vi "App - analyze RUS V6.vi"() -> ()   [LabVIEW 2015] (continued)
"Magn Field(T)"=0.0}, {"temperature"=56.174, "lorentzian"={"Amplitude"=0.0, "omega(0)"=0.0, "Gamma"=0.0, "phase"=0.0, "Q"=0.0, "Norm  Ampl"=0.0, "z (inf)"=0.0+0.0i, "4corners"={"z (-pi/2)"=0.0+0.0i, "z(inf)"=0.0+0.0i, "z (pi/2)"=0.0+0.0i, "z center"=0.0+0.0i, "z(0)"=0.0+0.0i, "radius"=0.0}}, "timestamp(min)"=1312.25, "timestamp"=timestamp(3493806556 s since 1904-01-01), "Magn Field(T)"=0.0}, {"temperature"=56.114, "lorentzian"={"Amplitude"=0.0, "omega(0)"=0.0, "Gamma"=0.0, "phase"=0.0, "Q"=0.0, "Norm  Ampl"=0.0, "z (inf)"=0.0+0.0i, "4corners"={"z (-pi/2)"=0.0+0.0i, "z(inf)"=0.0+0.0i, "z (pi/2)"=0.0+0.0i, "z center"=0.0+0.0i, "z(0)"=0.0+0.0i, "radius"=0.0}}, "timestamp(min)"=1313.5666666701436, "timestamp"=timestamp(3493806635 s since 1904-01-01), "Magn Field(T)"=0.0}, {"temperature"=56.051, "lorentzian"={"Amplitude"=0.0, "omega(0)"=0.0, "Gamma"=0.0, "phase"=0.0, "Q"=0.0, "Norm  Ampl"=0.0, "z (inf)"=0.0+0.0i, "4corners"={"z (-pi/2)"=0.0+0.0i, "z(inf)"=0.0+0.0i, "z (pi/2)"=0.0+0.0i, "z center"=0.0+0.0i, "z(0)"=0.0+0.0i, "radius"=0.0}}, "timestamp(min)"=1314.8833333328366, "timestamp"=timestamp(3493806714 s since 1904-01-01), "Magn Field(T)"=0.0}, {"temperature"=55.989, "lorentzian"={"Amplitude"=0.0, "omega(0)"=0.0, "Gamma"=0.0, "phase"=0.0, "Q"=0.0, "Norm  Ampl"=0.0, "z (inf)"=0.0+0.0i, "4corners"={"z (-pi/2)"=0.0+0.0i, "z(inf)"=0.0+0.0i, "z (pi/2)"=0.0+0.0i, "z center"=0.0+0.0i, "z(0)"=0.0+0.0i, "radius"=0.0}}, "timestamp(min)"=1316.2166666686535, "timestamp"=timestamp(3493806794 s since 1904-01-01), "Magn Field(T)"=0.0}, {"temperature"=55.93, "lorentzian"={"Amplitude"=0.0, "omega(0)"=0.0, "Gamma"=0.0, "phase"=0.0, "Q"=0.0, "Norm  Ampl"=0.0, "z (inf)"=0.0+0.0i, "4corners"={"z (-pi/2)"=0.0+0.0i, "z(inf)"=0.0+0.0i, "z (pi/2)"=0.0+0.0i, "z center"=0.0+0.0i, "z(0)"=0.0+0.0i, "radius"=0.0}}, "timestamp(min)"=1317.5333333313465, "timestamp"=timestamp(3493806873 s since 1904-01-01), "Magn Field(T)"=0.0}, {"temperature"=55.865, "lorentzian"={"Amplitude"=0.0, "omega(0)"=0.0, "Gamma"=0.0, "phase"=0.0, "Q"=0.0, "Norm  Ampl"=0.0, "z (inf)"=0.0+0.0i, "4corners"={"z (-pi/2)"=0.0+0.0i, "z(inf)"=0.0+0.0i, "z (pi/2)"=0.0+0.0i, "z center"=0.0+0.0i, "z(0)"=0.0+0.0i, "radius"=0.0}}, "timestamp(min)"=1318.8500000014901, "timestamp"=timestamp(3493806952 s since 1904-01-01), "Magn Field(T)"=0.0}, {"temperature"=55.805, "lorentzian"={"Amplitude"=0.0, "omega(0)"=0.0, "Gamma"=0.0, "phase"=0.0, "Q"=0.0, "Norm  Ampl"=0.0, "z (inf)"=0.0+0.0i, "4corners"={"z (-pi/2)"=0.0+0.0i, "z(inf)"=0.0+0.0i, "z (pi/2)"=0.0+0.0i, "z center"=0.0+0.0i, "z(0)"=0.0+0.0i, "radius"=0.0}}, "timestamp(min)"=1320.183333337307, "timestamp"=timestamp(3493807032 s since 1904-01-01), "Magn Field(T)"=0.0}, {"temperature"=55.744, "lorentzian"={"Amplitude"=0.0, "omega(0)"=0.0, "Gamma"=0.0, "phase"=0.0, "Q"=0.0, "Norm  Ampl"=0.0, "z (inf)"=0.0+0.0i, "4corners"={"z (-pi/2)"=0.0+0.0i, "z(inf)"=0.0+0.0i, "z (pi/2)"=0.0+0.0i, "z center"=0.0+0.0i, "z(0)"=0.0+0.0i, "radius"=0.0}}, "timestamp(min)"=1321.5, "timestamp"=timestamp(3493807111 s since 1904-01-01), "Magn Field(T)"=0.0}, {"temperature"=55.681, "lorentzian"={"Amplitude"=0.0, "omega(0)"=0.0, "Gamma"=0.0, "phase"=0.0, "Q"=0.0, "Norm  Ampl"=0.0, "z (inf)"=0.0+0.0i, "4corners"={"z (-pi/2)"=0.0+0.0i, "z(inf)"=0.0+0.0i, "z (pi/2)"=0.0+0.0i, "z center"=0.0+0.0i, "z(0)"=0.0+0.0i, "radius"=0.0}}, "timestamp(min)"=1322.8333333358169, "timestamp"=timestamp(3493807191 s since 1904-01-01), "Magn Field(T)"=0.0}, {"temperature"=55.622, "lorentzian"={"Amplitude"=0.0, "omega(0)"=0.0, "Gamma"=0.0, "phase"=0.0, "Q"=0.0, "Norm  Ampl"=0.0, "z (inf)"=0.0+0.0i, "4corners"={"z (-pi/2)"=0.0+0.0i, "z(inf)"=0.0+0.0i, "z (pi/2)"=0.0+0.0i, "z center"=0.0+0.0i, "z(0)"=0.0+0.0i, "radius"=0.0}}, "timestamp(min)"=1324.1499999985099, "timestamp"=timestamp(3493807270 s since 1904-01-01), "Magn Field(T)"=0.0}, {"temperature"=55.56, "lorentzian"={"Amplitude"=0.0, "omega(0)"=0.0, "Gamma"=0.0, "phase"=0.0, "Q"=0.0, "Norm  Ampl"=0.0, "z (inf)"=0.0+0.0i, "4corners"={"z (-pi/2)"=0.0+0.0i, "z(inf)"=0.0+0.0i, "z (pi/2)"=0.0+0.0i, "z center"=0.0+0.0i, "z(0)"=0.0+0.0i, "radius"=0.0}}, "timestamp(min)"=1325.4666666686535, "timestamp"=timestamp(3493807349 s since 1904-01-01), "Magn Field(T)"=0.0}, {"temperature"=55.498, "lorentzian"={"Amplitude"=0.0, "omega(0)"=0.0, "Gamma"=0.0, "phase"=0.0, "Q"=0.0, "Norm  Ampl"=0.0, "z (inf)"=0.0+0.0i, "4corners"={"z (-pi/2)"=0.0+0.0i, "z(inf)"=0.0+0.0i, "z (pi/2)"=0.0+0.0i, "z center"=0.0+0.0i, "z(0)"=0.0+0.0i, "radius"=0.0}}, "timestamp(min)"=1326.8000000044703, "timestamp"=timestamp(3493807429 s since 1904-01-01), "Magn Field(T)"=0.0}, {"temperature"=55.437, "lorentzian"={"Amplitude"=0.0, "omega(0)"=0.0, "Gamma"=0.0, "phase"=0.0, "Q"=0.0, "Norm  Ampl"=0.0, "z (inf)"=0.0+0.0i, "4corners"={"z (-pi/2)"=0.0+0.0i, "z(inf)"=0.0+0.0i, "z (pi/2)"=0.0+0.0i, "z center"=0.0+0.0i, "z(0)"=0.0+0.0i, "radius"=0.0}}, "timestamp(min)"=1328.1166666671634, "timestamp"=timestamp(3493807508 s since 1904-01-01), "Magn Field(T)"=0.0}, {"temperature"=55.376, "lorentzian"={"Amplitude"=0.0, "omega(0)"=0.0, "Gamma"=0.0, "phase"=0.0, "Q"=0.0, "Norm  Ampl"=0.0, "z (inf)"=0.0+0.0i, "4corners"={"z (-pi/2)"=0.0+0.0i, "z(inf)"=0.0+0.0i, "z (pi/2)"=0.0+0.0i, "z center"=0.0+0.0i, "z(0)"=0.0+0.0i, "radius"=0.0}}, "timestamp(min)"=1329.433333337307, "timestamp"=timestamp(3493807587 s since 1904-01-01), "Magn Field(T)"=0.0}, {"temperature"=55.311, "lorentzian"={"Amplitude"=0.0, "omega(0)"=0.0, "Gamma"=0.0, "phase"=0.0, "Q"=0.0, "Norm  Ampl"=0.0, "z (inf)"=0.0+0.0i, "4corners"={"z (-pi/2)"=0.0+0.0i, "z(inf)"=0.0+0.0i, "z (pi/2)"=0.0+0.0i, "z center"=0.0+0.0i, "z(0)"=0.0+0.0i, "radius"=0.0}}, "timestamp(min)"=1330.7666666656733, "timestamp"=timestamp(3493807667 s since 1904-01-01), "Magn Field(T)"=0.0}, {"temperature"=55.252, "lorentzian"={"Amplitude"=0.0, "omega(0)"=0.0, "Gamma"=0.0, "phase"=0.0, "Q"=0.0, "Norm  Ampl"=0.0, "z (inf)"=0.0+0.0i, "4corners"={"z (-pi/2)"=0.0+0.0i, "z(inf)"=0.0+0.0i, "z (pi/2)"=0.0+0.0i, "z center"=0.0+0.0i, "z(0)"=0.0+0.0i, "radius"=0.0}}, "timestamp(min)"=1332.0833333358169, "timestamp"=timestamp(3493807746 s since 1904-01-01), "Magn Field(T)"=0.0}, {"temperature"=55.188, "lorentzian"={"Amplitude"=0.0, "omega(0)"=0.0, "Gamma"=0.0, "phase"=0.0, "Q"=0.0, "Norm  Ampl"=0.0, "z (inf)"=0.0+0.0i, "4corners"={"z (-pi/2)"=0.0+0.0i, "z(inf)"=0.0+0.0i, "z (pi/2)"=0.0+0.0i, "z center"=0.0+0.0i, "z(0)"=0.0+0.0i, "radius"=0.0}}, "timestamp(min)"=1333.3999999985099, "timestamp"=timestamp(3493807825 s since 1904-01-01), "Magn Field(T)"=0.0}, {"temperature"=55.128, "lorentzian"={"Amplitude"=0.0, "omega(0)"=0.0, "Gamma"=0.0, "phase"=0.0, "Q"=0.0, "Norm  Ampl"=0.0, "z (inf)"=0.0+0.0i, "4corners"={"z (-pi/2)"=0.0+0.0i, "z(inf)"=0.0+0.0i, "z (pi/2)"=0.0+0.0i, "z center"=0.0+0.0i, "z(0)"=0.0+0.0i, "radius"=0.0}}, "timestamp(min)"=1334.7333333343267, "timestamp"=timestamp(3493807905 s since 1904-01-01), "Magn Field(T)"=0.0}, {"temperature"=55.063, "lorentzian"={"Amplitude"=0.0, "omega(0)"=0.0, "Gamma"=0.0, "phase"=0.0, "Q"=0.0, "Norm  Ampl"=0.0, "z (inf)"=0.0+0.0i, "4corners"={"z (-pi/2)"=0.0+0.0i, "z(inf)"=0.0+0.0i, "z (pi/2)"=0.0+0.0i, "z center"=0.0+0.0i, "z(0)"=0.0+0.0i, "radius"=0.0}}, "timestamp(min)"=1336.0500000044703, "timestamp"=timestamp(3493807984 s since 1904-01-01), "Magn Field(T)"=0.0}, {"temperature"=54.998, "lorentzian"={"Amplitude"=0.0, "omega(0)"=0.0, "Gamma"=0.0, "phase"=0.0, "Q"=0.0, "Norm  Ampl"=0.0, "z (inf)"=0.0+0.0i, "4corners"={"z (-pi/2)"=0.0+0.0i, "z(inf)"=0.0+0.0i, "z (pi/2)"=0.0+0.0i, "z center"=0.0+0.0i, "z(0)"=0.0+0.0i, "radius"=0.0}}, "timestamp(min)"=1337.3666666671634, "timestamp"=timestamp(3493808063 s since 1904-01-01), "Magn Field(T)"=0.0}, {"temperature"=54.938, "lorentzian"={"Amplitude"=0.0, "omega(0)"=0.0, "Gamma"=0.0, "phase"=0.0, "Q"=0.0, "Norm  Ampl"=0.0, "z (inf)"=0.0+0.0i, "4corners"={"z (-pi/2)"=0.0+0.0i, "z(inf)"=0.0+0.0i, "z (pi/2)"=0.0+0.0i, "z center"=0.0+0.0i, "z(0)"=0.0+0.0i, "radius"=0.0}}, "timestamp(min)"=1338.7000000029802, "timestamp"=timestamp(3493808143 s since 1904-01-01), "Magn Field(T)"=0.0}, {"temperature"=54.879, "lorentzian"={"Amplitude"=0.0, "omega(0)"=0.0, "Gamma"=0.0, "phase"=0.0, "Q"=0.0, "Norm  Ampl"=0.0, "z (inf)"=0.0+0.0i, "4corners"={"z (-pi/2)"=0.0+0.0i, "z(inf)"=0.0+0.0i, "z (pi/2)"=0.0+0.0i, "z center"=0.0+0.0i, "z(0)"=0.0+0.0i, "radius"=0.0}}, "timestamp(min)"=1340.0166666656733, "timestamp"=timestamp(3493808222 s since 1904-01-01), "Magn Field(T)"=0.0}, {"temperature"=54.816, "lorentzian"={"Amplitude"=0.0, "omega(0)"=0.0, "Gamma"=0.0, "phase"=0.0, "Q"=0.0, "Norm  Ampl"=0.0, "z (inf)"=0.0+0.0i, "4corners"={"z (-pi/2)"=0.0+0.0i, "z(inf)"=0.0+0.0i, "z (pi/2)"=0.0+0.0i, "z center"=0.0+0.0i, "z(0)"=0.0+0.0i, "radius"=0.0}}, "timestamp(min)"=1341.3333333358169, "timestamp"=timestamp(3493808301 s since 1904-01-01), "Magn Field(T)"=0.0}, {"temperature"=54.752, "lorentzian"={"Amplitude"=0.0, "omega(0)"=0.0, "Gamma"=0.0, "phase"=0.0, "Q"=0.0, "Norm  Ampl"=0.0, "z (inf)"=0.0+0.0i, "4corners"={"z (-pi/2)"=0.0+0.0i, "z(inf)"=0.0+0.0i, "z (pi/2)"=0.0+0.0i, "z center"=0.0+0.0i, "z(0)"=0.0+0.0i, "radius"=0.0}}, "timestamp(min)"=1342.6666666641831, "timestamp"=timestamp(3493808381 s since 1904-01-01), "Magn Field(T)"=0.0}, {"temperature"=54.691, "lorentzian"={"Amplitude"=0.0, "omega(0)"=0.0, "Gamma"=0.0, "phase"=0.0, "Q"=0.0, "Norm  Ampl"=0.0, "z (inf)"=0.0+0.0i, "4corners"={"z (-pi/2)"=0.0+0.0i, "z(inf)"=0.0+0.0i, "z (pi/2)"=0.0+0.0i, "z center"=0.0+0.0i, "z(0)"=0.0+0.0i, "radius"=0.0}}, "timestamp(min)"=1343.9833333343267, "timestamp"=timestamp(3493808460 s since 1904-01-01), "Magn Field(T)"=0.0}, {"temperature"=54.628, "lorentzian"={"Amplitude"=0.0, "omega(0)"=0.0, "Gamma"=0.0, "phase"=0.0, "Q"=0.0, "Norm  Ampl"=0.0, "z (inf)"=0.0+0.0i, "4corners"={"z (-pi/2)"=0.0+0.0i, "z(inf)"=0.0+0.0i, "z (pi/2)"=0.0+0.0i, "z center"=0.0+0.0i, "z(0)"=0.0+0.0i, "radius"=0.0}}, "timestamp(min)"=1345.3000000044703, "timestamp"=timestamp(3493808539 s since 1904-01-01), "Magn Field(T)"=0.0}, {"temperature"=54.564, "lorentzian"={"Amplitude"=0.0, "omega(0)"=0.0, "Gamma"=0.0, "phase"=0.0, "Q"=0.0, "Norm  Ampl"=0.0, "z (inf)"=0.0+0.0i, "4corners"={"z (-pi/2)"=0.0+0.0i, "z(inf)"=0.0+0.0i, "z (pi/2)"=0.0+0.0i, "z center"=0.0+0.0i, "z(0)"=0.0+0.0i, "radius"=0.0}}, "timestamp(min)"=1346.6333333328366, "timestamp"=timestamp(3493808619 s since 1904-01-01), "Magn Field(T)"=0.0}, {"temperature"=54.505, "lorentzian"={"Amplitude"=0.0, "omega(0)"=0.0, "Gamma"=0.0, "phase"=0.0, "Q"=0.0, "Norm  Ampl"=0.0, "z (inf)"=0.0+0.0i, "4corners"={"z (-pi/2)"=0.0+0.0i, "z(inf)"=0.0+0.0i, "z (pi/2)"=0.0+0.0i, "z center"=0.0+0.0i, "z(0)"=0.0+0.0i, "radius"=0.0}}, "timestamp(min)"=1347.9500000029802, "timestamp"=timestamp(3493808698 s since 1904-01-01), "Magn Field(T)"=0.0}, {"temperature"=54.44, "lorentzian"={"Amplitude"=0.0, "omega(0)"=0.0, "Gamma"=0.0, "phase"=0.0, "Q"=0.0, "Norm  Ampl"=0.0, "z (inf)"=0.0+0.0i, "4corners"={"z (-pi/2)"=0.0+0.0i, "z(inf)"=0.0+0.0i, "z (pi/2)"=0.0+0.0i, "z center"=0.0+0.0i, "z(0)"=0.0+0.0i, "radius"=0.0}}, "timestamp(min)"=1349.2833333313465, "timestamp"=timestamp(3493808778 s since 1904-01-01), "Magn Field(T)"=0.0}, {"temperature"=54.375, "lorentzian"={"Amplitude"=0.0, "omega(0)"=0.0, "Gamma"=0.0, "phase"=0.0, "Q"=0.0, "Norm  Ampl"=0.0, "z (inf)"=0.0+0.0i, "4corners"={"z (-pi/2)"=0.0+0.0i, "z(inf)"=0.0+0.0i, "z (pi/2)"=0.0+0.0i, "z center"=0.0+0.0i, "z(0)"=0.0+0.0i, "radius"=0.0}}, "timestamp(min)"=1350.6000000014901, "timestamp"=timestamp(3493808857 s since 1904-01-01), "Magn Field(T)"=0.0}, {"temperature"=54.316, "lorentzian"={"Amplitude"=0.0, "omega(0)"=0.0, "Gamma"=0.0, "phase"=0.0, "Q"=0.0, "Norm  Ampl"=0.0, "z (inf)"=0.0+0.0i, "4corners"={"z (-pi/2)"=0.0+0.0i, "z(inf)"=0.0+0.0i, "z (pi/2)"=0.0+0.0i, "z center"=0.0+0.0i, "z(0)"=0.0+0.0i, "radius"=0.0}}, "timestamp(min)"=1351.9166666641831, "timestamp"=timestamp(3493808936 s since 1904-01-01), "Magn Field(T)"=0.0}, {"temperature"=54.252, "lorentzian"={"Amplitude"=0.0, "omega(0)"=0.0, "Gamma"=0.0, "phase"=0.0, "Q"=0.0, "Norm  Ampl"=0.0, "z (inf)"=0.0+0.0i, "4corners"={"z (-pi/2)"=0.0+0.0i, "z(inf)"=0.0+0.0i, "z (pi/2)"=0.0+0.0i, "z center"=0.0+0.0i, "z(0)"=0.0+0.0i, "radius"=0.0}}, "timestamp(min)"=1353.25, "timestamp"=timestamp(3493809016 s since 1904-01-01), "Magn Field(T)"=0.0}, {"temperature"=54.191, "lorentzian"={"Amplitude"=0.0, "omega(0)"=0.0, "Gamma"=0.0, "phase"=0.0, "Q"=0.0, "Norm  Ampl"=0.0, "z (inf)"=0.0+0.0i, "4corners"={"z (-pi/2)"=0.0+0.0i, "z(inf)"=0.0+0.0i, "z (pi/2)"=0.0+0.0i, "z center"=0.0+0.0i, "z(0)"=0.0+0.0i, "radius"=0.0}}, "timestamp(min)"=1354.5666666701436, "timestamp"=timestamp(3493809095 s since 1904-01-01), "Magn Field(T)"=0.0}, {"temperature"=54.128, "lorentzian"={"Amplitude"=0.0, "omega(0)"=0.0, "Gamma"=0.0, "phase"=0.0, "Q"=0.0, "Norm  Ampl"=0.0, "z (inf)"=0.0+0.0i, "4corners"={"z (-pi/2)"=0.0+0.0i, "z(inf)"=0.0+0.0i, "z (pi/2)"=0.0+0.0i, "z center"=0.0+0.0i, "z(0)"=0.0+0.0i, "radius"=0.0}}, "timestamp(min)"=1355.8833333328366, "timestamp"=timestamp(3493809174 s since 1904-01-01), "Magn Field(T)"=0.0}, {"temperature"=54.064, "lorentzian"={"Amplitude"=0.0, "omega(0)"=0.0, "Gamma"=0.0, "phase"=0.0, "Q"=0.0, "Norm  Ampl"=0.0, "z (inf)"=0.0+0.0i, "4corners"={"z (-pi/2)"=0.0+0.0i, "z(inf)"=0.0+0.0i, "z (pi/2)"=0.0+0.0i, "z center"=0.0+0.0i, "z(0)"=0.0+0.0i, "radius"=0.0}}, "timestamp(min)"=1357.2166666686535, "timestamp"=timestamp(3493809254 s since 1904-01-01), "Magn Field(T)"=0.0}, {"temperature"=54.004, "lorentzian"={"Amplitude"=0.0, "omega(0)"=0.0, "Gamma"=0.0, "phase"=0.0, "Q"=0.0, "Norm  Ampl"=0.0, "z (inf)"=0.0+0.0i, "4corners"={"z (-pi/2)"=0.0+0.0i, "z(inf)"=0.0+0.0i, "z (pi/2)"=0.0+0.0i, "z center"=0.0+0.0i, "z(0)"=0.0+0.0i, "radius"=0.0}}, "timestamp(min)"=1358.5333333313465, "timestamp"=timestamp(3493809333 s since 1904-01-01), "Magn Field(T)"=0.0}, {"temperature"=53.936, "lorentzian"={"Amplitude"=0.0, "omega(0)"=0.0, "Gamma"=0.0, "phase"=0.0, "Q"=0.0, "Norm  Ampl"=0.0, "z (inf)"=0.0+0.0i, "4corners"={"z (-pi/2)"=0.0+0.0i, "z(inf)"=0.0+0.0i, "z (pi/2)"=0.0+0.0i, "z center"=0.0+0.0i, "z(0)"=0.0+0.0i, "radius"=0.0}}, "timestamp(min)"=1359.8666666671634, "timestamp"=timestamp(3493809413 s since 1904-01-01), "Magn Field(T)"=0.0}, {"temperature"=53.874, "lorentzian"={"Amplitude"=0.0, "omega(0)"=0.0, "Gamma"=0.0, "phase"=0.0, "Q"=0.0, "Norm  Ampl"=0.0, "z (inf)"=0.0+0.0i, "4corners"={"z (-pi/2)"=0.0+0.0i, "z(inf)"=0.0+0.0i, "z (pi/2)"=0.0+0.0i, "z center"=0.0+0.0i, "z(0)"=0.0+0.0i, "radius"=0.0}}, "timestamp(min)"=1361.183333337307, "timestamp"=timestamp(3493809492 s since 1904-01-01), "Magn Field(T)"=0.0}, {"temperature"=53.813, "lorentzian"={"Amplitude"=0.0, "omega(0)"=0.0, "Gamma"=0.0, "phase"=0.0, "Q"=0.0, "Norm  Ampl"=0.0, "z (inf)"=0.0+0.0i, "4corners"={"z (-pi/2)"=0.0+0.0i, "z(inf)"=0.0+0.0i, "z (pi/2)"=0.0+0.0i, "z center"=0.0+0.0i, "z(0)"=0.0+0.0i, "radius"=0.0}}, "timestamp(min)"=1362.5, "timestamp"=timestamp(3493809571 s since 1904-01-01), "Magn Field(T)"=0.0}, {"temperature"=53.746, "lorentzian"={"Amplitude"=0.0, "omega(0)"=0.0, "Gamma"=0.0, "phase"=0.0, "Q"=0.0, "Norm  Ampl"=0.0, "z (inf)"=0.0+0.0i, "4corners"={"z (-pi/2)"=0.0+0.0i, "z(inf)"=0.0+0.0i, "z (pi/2)"=0.0+0.0i, "z center"=0.0+0.0i, "z(0)"=0.0+0.0i, "radius"=0.0}}, "timestamp(min)"=1363.8333333358169, "timestamp"=timestamp(3493809651 s since 1904-01-01), "Magn Field(T)"=0.0}, {"temperature"=53.683, "lorentzian"={"Amplitude"=0.0, "omega(0)"=0.0, "Gamma"=0.0, "phase"=0.0, "Q"=0.0, "Norm  Ampl"=0.0, "z (inf)"=0.0+0.0i, "4corners"={"z (-pi/2)"=0.0+0.0i, "z(inf)"=0.0+0.0i, "z (pi/2)"=0.0+0.0i, "z center"=0.0+0.0i, "z(0)"=0.0+0.0i, "radius"=0.0}}, "timestamp(min)"=1365.1499999985099, "timestamp"=timestamp(3493809730 s since 1904-01-01), "Magn Field(T)"=0.0}, {"temperature"=53.622, "lorentzian"={"Amplitude"=0.0, "omega(0)"=0.0, "Gamma"=0.0, "phase"=0.0, "Q"=0.0, "Norm  Ampl"=0.0, "z (inf)"=0.0+0.0i, "4corners"={"z (-pi/2)"=0.0+0.0i, "z(inf)"=0.0+0.0i, "z (pi/2)"=0.0+0.0i, "z center"=0.0+0.0i, "z(0)"=0.0+0.0i, "radius"=0.0}}, "timestamp(min)"=1366.4666666686535, "timestamp"=timestamp(3493809809 s since 1904-01-01), "Magn Field(T)"=0.0}, {"temperature"=53.557, "lorentzian"={"Amplitude"=0.0, "omega(0)"=0.0, "Gamma"=0.0, "phase"=0.0, "Q"=0.0, "Norm  Ampl"=0.0, "z (inf)"=0.0+0.0i, "4corners"={"z (-pi/2)"=0.0+0.0i, "z(inf)"=0.0+0.0i, "z (pi/2)"=0.0+0.0i, "z center"=0.0+0.0i, "z(0)"=0.0+0.0i, "radius"=0.0}}, "timestamp(min)"=1367.8000000044703, "timestamp"=timestamp(3493809889 s since 1904-01-01), "Magn Field(T)"=0.0}, {"temperature"=53.492, "lorentzian"={"Amplitude"=0.0, "omega(0)"=0.0, "Gamma"=0.0, "phase"=0.0, "Q"=0.0, "Norm  Ampl"=0.0, "z (inf)"=0.0+0.0i, "4corners"={"z (-pi/2)"=0.0+0.0i, "z(inf)"=0.0+0.0i, "z (pi/2)"=0.0+0.0i, "z center"=0.0+0.0i, "z(0)"=0.0+0.0i, "radius"=0.0}}, "timestamp(min)"=1369.1166666671634, "timestamp"=timestamp(3493809968 s since 1904-01-01), "Magn Field(T)"=0.0}, {"temperature"=53.431, "lorentzian"={"Amplitude"=0.0, "omega(0)"=0.0, "Gamma"=0.0, "phase"=0.0, "Q"=0.0, "Norm  Ampl"=0.0, "z (inf)"=0.0+0.0i, "4corners"={"z (-pi/2)"=0.0+0.0i, "z(inf)"=0.0+0.0i, "z (pi/2)"=0.0+0.0i, "z center"=0.0+0.0i, "z(0)"=0.0+0.0i, "radius"=0.0}}, "timestamp(min)"=1370.4500000029802, "timestamp"=timestamp(3493810048 s since 1904-01-01), "Magn Field(T)"=0.0}, {"temperature"=53.368, "lorentzian"={"Amplitude"=0.0, "omega(0)"=0.0, "Gamma"=0.0, "phase"=0.0, "Q"=0.0, "Norm  Ampl"=0.0, "z (inf)"=0.0+0.0i, "4corners"={"z (-pi/2)"=0.0+0.0i, "z(inf)"=0.0+0.0i, "z (pi/2)"=0.0+0.0i, "z center"=0.0+0.0i, "z(0)"=0.0+0.0i, "radius"=0.0}}, "timestamp(min)"=1371.7666666656733, "timestamp"=timestamp(3493810127 s since 1904-01-01), "Magn Field(T)"=0.0}, {"temperature"=53.304, "lorentzian"={"Amplitude"=0.0, "omega(0)"=0.0, "Gamma"=0.0, "phase"=0.0, "Q"=0.0, "Norm  Ampl"=0.0, "z (inf)"=0.0+0.0i, "4corners"={"z (-pi/2)"=0.0+0.0i, "z(inf)"=0.0+0.0i, "z (pi/2)"=0.0+0.0i, "z center"=0.0+0.0i, "z(0)"=0.0+0.0i, "radius"=0.0}}, "timestamp(min)"=1373.0833333358169, "timestamp"=timestamp(3493810206 s since 1904-01-01), "Magn Field(T)"=0.0}, {"temperature"=53.234, "lorentzian"={"Amplitude"=0.0, "omega(0)"=0.0, "Gamma"=0.0, "phase"=0.0, "Q"=0.0, "Norm  Ampl"=0.0, "z (inf)"=0.0+0.0i, "4corners"={"z (-pi/2)"=0.0+0.0i, "z(inf)"=0.0+0.0i, "z (pi/2)"=0.0+0.0i, "z center"=0.0+0.0i, "z(0)"=0.0+0.0i, "radius"=0.0}}, "timestamp(min)"=1374.4166666641831, "timestamp"=timestamp(3493810286 s since 1904-01-01), "Magn Field(T)"=0.0}, {"temperature"=53.178, "lorentzian"={"Amplitude"=0.0, "omega(0)"=0.0, "Gamma"=0.0, "phase"=0.0, "Q"=0.0, "Norm  Ampl"=0.0, "z (inf)"=0.0+0.0i, "4corners"={"z (-pi/2)"=0.0+0.0i, "z(inf)"=0.0+0.0i, "z (pi/2)"=0.0+0.0i, "z center"=0.0+0.0i, "z(0)"=0.0+0.0i, "radius"=0.0}}, "timestamp(min)"=1375.7333333343267, "timestamp"=timestamp(3493810365 s since 1904-01-01), "Magn Field(T)"=0.0}, {"temperature"=53.112, "lorentzian"={"Amplitude"=0.0, "omega(0)"=0.0, "Gamma"=0.0, "phase"=0.0, "Q"=0.0, "Norm  Ampl"=0.0, "z (inf)"=0.0+0.0i, "4corners"={"z (-pi/2)"=0.0+0.0i, "z(inf)"=0.0+0.0i, "z (pi/2)"=0.0+0.0i, "z center"=0.0+0.0i, "z(0)"=0.0+0.0i, "radius"=0.0}}, "timestamp(min)"=1377.0500000044703, "timestamp"=timestamp(3493810444 s since 1904-01-01), "Magn Field(T)"=0.0}, {"temperature"=53.046, "lorentzian"={"Amplitude"=0.0, "omega(0)"=0.0, "Gamma"=0.0, "phase"=0.0, "Q"=0.0, "Norm  Ampl"=0.0, "z (inf)"=0.0+0.0i, "4corners"={"z (-pi/2)"=0.0+0.0i, "z(inf)"=0.0+0.0i, "z (pi/2)"=0.0+0.0i, "z center"=0.0+0.0i, "z(0)"=0.0+0.0i, "radius"=0.0}}, "timestamp(min)"=1378.3833333328366, "timestamp"=timestamp(3493810524 s since 1904-01-01), "Magn Field(T)"=0.0}, {"temperature"=52.981, "lorentzian"={"Amplitude"=0.0, "omega(0)"=0.0, "Gamma"=0.0, "phase"=0.0, "Q"=0.0, "Norm  Ampl"=0.0, "z (inf)"=0.0+0.0i, "4corners"={"z (-pi/2)"=0.0+0.0i, "z(inf)"=0.0+0.0i, "z (pi/2)"=0.0+0.0i, "z center"=0.0+0.0i, "z(0)"=0.0+0.0i, "radius"=0.0}}, "timestamp(min)"=1379.7000000029802, "timestamp"=timestamp(3493810603 s since 1904-01-01), "Magn Field(T)"=0.0}, {"temperature"=52.922, "lorentzian"={"Amplitude"=0.0, "omega(0)"=0.0, "Gamma"=0.0, "phase"=0.0, "Q"=0.0, "Norm  Ampl"=0.0, "z (inf)"=0.0+0.0i, "4corners"={"z (-pi/2)"=0.0+0.0i, "z(inf)"=0.0+0.0i, "z (pi/2)"=0.0+0.0i, "z center"=0.0+0.0i, "z(0)"=0.0+0.0i, "radius"=0.0}}, "timestamp(min)"=1381.0333333313465, "timestamp"=timestamp(3493810683 s since 1904-01-01), "Magn Field(T)"=0.0}, {"temperature"=52.856, "lorentzian"={"Amplitude"=0.0, "omega(0)"=0.0, "Gamma"=0.0, "phase"=0.0, "Q"=0.0, "Norm  Ampl"=0.0, "z (inf)"=0.0+0.0i, "4corners"={"z (-pi/2)"=0.0+0.0i, "z(inf)"=0.0+0.0i, "z (pi/2)"=0.0+0.0i, "z center"=0.0+0.0i, "z(0)"=0.0+0.0i, "radius"=0.0}}, "timestamp(min)"=1382.3500000014901, "timestamp"=timestamp(3493810762 s since 1904-01-01), "Magn Field(T)"=0.0}, {"temperature"=52.786, "lorentzian"={"Amplitude"=0.0, "omega(0)"=0.0, "Gamma"=0.0, "phase"=0.0, "Q"=0.0, "Norm  Ampl"=0.0, "z (inf)"=0.0+0.0i, "4corners"={"z (-pi/2)"=0.0+0.0i, "z(inf)"=0.0+0.0i, "z (pi/2)"=0.0+0.0i, "z center"=0.0+0.0i, "z(0)"=0.0+0.0i, "radius"=0.0}}, "timestamp(min)"=1383.6666666641831, "timestamp"=timestamp(3493810841 s since 1904-01-01), "Magn Field(T)"=0.0}, {"temperature"=52.726, "lorentzian"={"Amplitude"=0.0, "omega(0)"=0.0, "Gamma"=0.0, "phase"=0.0, "Q"=0.0, "Norm  Ampl"=0.0, "z (inf)"=0.0+0.0i, "4corners"={"z (-pi/2)"=0.0+0.0i, "z(inf)"=0.0+0.0i, "z (pi/2)"=0.0+0.0i, "z center"=0.0+0.0i, "z(0)"=0.0+0.0i, "radius"=0.0}}, "timestamp(min)"=1385.0, "timestamp"=timestamp(3493810921 s since 1904-01-01), "Magn Field(T)"=0.0}, {"temperature"=52.665, "lorentzian"={"Amplitude"=0.0, "omega(0)"=0.0, "Gamma"=0.0, "phase"=0.0, "Q"=0.0, "Norm  Ampl"=0.0, "z (inf)"=0.0+0.0i, "4corners"={"z (-pi/2)"=0.0+0.0i, "z(inf)"=0.0+0.0i, "z (pi/2)"=0.0+0.0i, "z center"=0.0+0.0i, "z(0)"=0.0+0.0i, "radius"=0.0}}, "timestamp(min)"=1386.3166666701436, "timestamp"=timestamp(3493811000 s since 1904-01-01), "Magn Field(T)"=0.0}, {"temperature"=52.593, "lorentzian"={"Amplitude"=0.0, "omega(0)"=0.0, "Gamma"=0.0, "phase"=0.0, "Q"=0.0, "Norm  Ampl"=0.0, "z (inf)"=0.0+0.0i, "4corners"={"z (-pi/2)"=0.0+0.0i, "z(inf)"=0.0+0.0i, "z (pi/2)"=0.0+0.0i, "z center"=0.0+0.0i, "z(0)"=0.0+0.0i, "radius"=0.0}}, "timestamp(min)"=1387.6333333328366, "timestamp"=timestamp(3493811079 s since 1904-01-01), "Magn Field(T)"=0.0}, {"temperature"=52.53, "lorentzian"={"Amplitude"=0.0, "omega(0)"=0.0, "Gamma"=0.0, "phase"=0.0, "Q"=0.0, "Norm  Ampl"=0.0, "z (inf)"=0.0+0.0i, "4corners"={"z (-pi/2)"=0.0+0.0i, "z(inf)"=0.0+0.0i, "z (pi/2)"=0.0+0.0i, "z center"=0.0+0.0i, "z(0)"=0.0+0.0i, "radius"=0.0}}, "timestamp(min)"=1388.9666666686535, "timestamp"=timestamp(3493811159 s since 1904-01-01), "Magn Field(T)"=0.0}, {"temperature"=52.467, "lorentzian"={"Amplitude"=0.0, "omega(0)"=0.0, "Gamma"=0.0, "phase"=0.0, "Q"=0.0, "Norm  Ampl"=0.0, "z (inf)"=0.0+0.0i, "4corners"={"z (-pi/2)"=0.0+0.0i, "z(inf)"=0.0+0.0i, "z (pi/2)"=0.0+0.0i, "z center"=0.0+0.0i, "z(0)"=0.0+0.0i, "radius"=0.0}}, "timestamp(min)"=1390.2833333313465, "timestamp"=timestamp(3493811238 s since 1904-01-01), "Magn Field(T)"=0.0}, {"temperature"=52.405, "lorentzian"={"Amplitude"=0.0, "omega(0)"=0.0, "Gamma"=0.0, "phase"=0.0, "Q"=0.0, "Norm  Ampl"=0.0, "z (inf)"=0.0+0.0i, "4corners"={"z (-pi/2)"=0.0+0.0i, "z(inf)"=0.0+0.0i, "z (pi/2)"=0.0+0.0i, "z center"=0.0+0.0i, "z(0)"=0.0+0.0i, "radius"=0.0}}, "timestamp(min)"=1391.6166666671634, "timestamp"=timestamp(3493811318 s since 1904-01-01), "Magn Field(T)"=0.0}, {"temperature"=52.337, "lorentzian"={"Amplitude"=0.0, "omega(0)"=0.0, "Gamma"=0.0, "phase"=0.0, "Q"=0.0, "Norm  Ampl"=0.0, "z (inf)"=0.0+0.0i, "4corners"={"z (-pi/2)"=0.0+0.0i, "z(inf)"=0.0+0.0i, "z (pi/2)"=0.0+0.0i, "z center"=0.0+0.0i, "z(0)"=0.0+0.0i, "radius"=0.0}}, "timestamp(min)"=1392.933333337307, "timestamp"=timestamp(3493811397 s since 1904-01-01), "Magn Field(T)"=0.0}, {"temperature"=52.27, "lorentzian"={"Amplitude"=0.0, "omega(0)"=0.0, "Gamma"=0.0, "phase"=0.0, "Q"=0.0, "Norm  Ampl"=0.0, "z (inf)"=0.0+0.0i, "4corners"={"z (-pi/2)"=0.0+0.0i, "z(inf)"=0.0+0.0i, "z (pi/2)"=0.0+0.0i, "z center"=0.0+0.0i, "z(0)"=0.0+0.0i, "radius"=0.0}}, "timestamp(min)"=1394.25, "timestamp"=timestamp(3493811476 s since 1904-01-01), "Magn Field(T)"=0.0}, {"temperature"=52.209, "lorentzian"={"Amplitude"=0.0, "omega(0)"=0.0, "Gamma"=0.0, "phase"=0.0, "Q"=0.0, "Norm  Ampl"=0.0, "z (inf)"=0.0+0.0i, "4corners"={"z (-pi/2)"=0.0+0.0i, "z(inf)"=0.0+0.0i, "z (pi/2)"=0.0+0.0i, "z center"=0.0+0.0i, "z(0)"=0.0+0.0i, "radius"=0.0}}, "timestamp(min)"=1395.5833333358169, "timestamp"=timestamp(3493811556 s since 1904-01-01), "Magn Field(T)"=0.0}, {"temperature"=52.142, "lorentzian"={"Amplitude"=0.0, "omega(0)"=0.0, "Gamma"=0.0, "phase"=0.0, "Q"=0.0, "Norm  Ampl"=0.0, "z (inf)"=0.0+0.0i, "4corners"={"z (-pi/2)"=0.0+0.0i, "z(inf)"=0.0+0.0i, "z (pi/2)"=0.0+0.0i, "z center"=0.0+0.0i, "z(0)"=0.0+0.0i, "radius"=0.0}}, "timestamp(min)"=1396.8999999985099, "timestamp"=timestamp(3493811635 s since 1904-01-01), "Magn Field(T)"=0.0}, {"temperature"=52.081, "lorentzian"={"Amplitude"=0.0, "omega(0)"=0.0, "Gamma"=0.0, "phase"=0.0, "Q"=0.0, "Norm  Ampl"=0.0, "z (inf)"=0.0+0.0i, "4corners"={"z (-pi/2)"=0.0+0.0i, "z(inf)"=0.0+0.0i, "z (pi/2)"=0.0+0.0i, "z center"=0.0+0.0i, "z(0)"=0.0+0.0i, "radius"=0.0}}, "timestamp(min)"=1398.2166666686535, "timestamp"=timestamp(3493811714 s since 1904-01-01), "Magn Field(T)"=0.0}, {"temperature"=52.015, "lorentzian"={"Amplitude"=0.0, "omega(0)"=0.0, "Gamma"=0.0, "phase"=0.0, "Q"=0.0, "Norm  Ampl"=0.0, "z (inf)"=0.0+0.0i, "4corners"={"z (-pi/2)"=0.0+0.0i, "z(inf)"=0.0+0.0i, "z (pi/2)"=0.0+0.0i, "z center"=0.0+0.0i, "z(0)"=0.0+0.0i, "radius"=0.0}}, "timestamp(min)"=1399.5500000044703, "timestamp"=timestamp(3493811794 s since 1904-01-01), "Magn Field(T)"=0.0}, {"temperature"=51.945, "lorentzian"={"Amplitude"=0.0, "omega(0)"=0.0, "Gamma"=0.0, "phase"=0.0, "Q"=0.0, "Norm  Ampl"=0.0, "z (inf)"=0.0+0.0i, "4corners"={"z (-pi/2)"=0.0+0.0i, "z(inf)"=0.0+0.0i, "z (pi/2)"=0.0+0.0i, "z center"=0.0+0.0i, "z(0)"=0.0+0.0i, "radius"=0.0}}, "timestamp(min)"=1400.8666666671634, "timestamp"=timestamp(3493811873 s since 1904-01-01), "Magn Field(T)"=0.0}, {"temperature"=51.883, "lorentzian"={"Amplitude"=0.0, "omega(0)"=0.0, "Gamma"=0.0, "phase"=0.0, "Q"=0.0, "Norm  Ampl"=0.0, "z (inf)"=0.0+0.0i, "4corners"={"z (-pi/2)"=0.0+0.0i, "z(inf)"=0.0+0.0i, "z (pi/2)"=0.0+0.0i, "z center"=0.0+0.0i, "z(0)"=0.0+0.0i, "radius"=0.0}}, "timestamp(min)"=1402.183333337307, "timestamp"=timestamp(3493811952 s since 1904-01-01), "Magn Field(T)"=0.0}, {"temperature"=51.82, "lorentzian"={"Amplitude"=0.0, "omega(0)"=0.0, "Gamma"=0.0, "phase"=0.0, "Q"=0.0, "Norm  Ampl"=0.0, "z (inf)"=0.0+0.0i, "4corners"={"z (-pi/2)"=0.0+0.0i, "z(inf)"=0.0+0.0i, "z (pi/2)"=0.0+0.0i, "z center"=0.0+0.0i, "z(0)"=0.0+0.0i, "radius"=0.0}}, "timestamp(min)"=1403.5166666656733, "timestamp"=timestamp(3493812032 s since 1904-01-01), "Magn Field(T)"=0.0}, {"temperature"=51.755, "lorentzian"={"Amplitude"=0.0, "omega(0)"=0.0, "Gamma"=0.0, "phase"=0.0, "Q"=0.0, "Norm  Ampl"=0.0, "z (inf)"=0.0+0.0i, "4corners"={"z (-pi/2)"=0.0+0.0i, "z(inf)"=0.0+0.0i, "z (pi/2)"=0.0+0.0i, "z center"=0.0+0.0i, "z(0)"=0.0+0.0i, "radius"=0.0}}, "timestamp(min)"=1404.8333333358169, "timestamp"=timestamp(3493812111 s since 1904-01-01), "Magn Field(T)"=0.0}, {"temperature"=51.682, "lorentzian"={"Amplitude"=0.0, "omega(0)"=0.0, "Gamma"=0.0, "phase"=0.0, "Q"=0.0, "Norm  Ampl"=0.0, "z (inf)"=0.0+0.0i, "4corners"={"z (-pi/2)"=0.0+0.0i, "z(inf)"=0.0+0.0i, "z (pi/2)"=0.0+0.0i, "z center"=0.0+0.0i, "z(0)"=0.0+0.0i, "radius"=0.0}}, "timestamp(min)"=1406.1666666641831, "timestamp"=timestamp(3493812191 s since 1904-01-01), "Magn Field(T)"=0.0}, {"temperature"=51.621, "lorentzian"={"Amplitude"=0.0, "omega(0)"=0.0, "Gamma"=0.0, "phase"=0.0, "Q"=0.0, "Norm  Ampl"=0.0, "z (inf)"=0.0+0.0i, "4corners"={"z (-pi/2)"=0.0+0.0i, "z(inf)"=0.0+0.0i, "z (pi/2)"=0.0+0.0i, "z center"=0.0+0.0i, "z(0)"=0.0+0.0i, "radius"=0.0}}, "timestamp(min)"=1407.4833333343267, "timestamp"=timestamp(3493812270 s since 1904-01-01), "Magn Field(T)"=0.0}, {"temperature"=51.556, "lorentzian"={"Amplitude"=0.0, "omega(0)"=0.0, "Gamma"=0.0, "phase"=0.0, "Q"=0.0, "Norm  Ampl"=0.0, "z (inf)"=0.0+0.0i, "4corners"={"z (-pi/2)"=0.0+0.0i, "z(inf)"=0.0+0.0i, "z (pi/2)"=0.0+0.0i, "z center"=0.0+0.0i, "z(0)"=0.0+0.0i, "radius"=0.0}}, "timestamp(min)"=1408.8000000044703, "timestamp"=timestamp(3493812349 s since 1904-01-01), "Magn Field(T)"=0.0}, {"temperature"=51.489, "lorentzian"={"Amplitude"=0.0, "omega(0)"=0.0, "Gamma"=0.0, "phase"=0.0, "Q"=0.0, "Norm  Ampl"=0.0, "z (inf)"=0.0+0.0i, "4corners"={"z (-pi/2)"=0.0+0.0i, "z(inf)"=0.0+0.0i, "z (pi/2)"=0.0+0.0i, "z center"=0.0+0.0i, "z(0)"=0.0+0.0i, "radius"=0.0}}, "timestamp(min)"=1410.1333333328366, "timestamp"=timestamp(3493812429 s since 1904-01-01), "Magn Field(T)"=0.0}, {"temperature"=51.422, "lorentzian"={"Amplitude"=0.0, "omega(0)"=0.0, "Gamma"=0.0, "phase"=0.0, "Q"=0.0, "Norm  Ampl"=0.0, "z (inf)"=0.0+0.0i, "4corners"={"z (-pi/2)"=0.0+0.0i, "z(inf)"=0.0+0.0i, "z (pi/2)"=0.0+0.0i, "z center"=0.0+0.0i, "z(0)"=0.0+0.0i, "radius"=0.0}}, "timestamp(min)"=1411.4500000029802, "timestamp"=timestamp(3493812508 s since 1904-01-01), "Magn Field(T)"=0.0}, {"temperature"=51.358, "lorentzian"={"Amplitude"=0.0, "omega(0)"=0.0, "Gamma"=0.0, "phase"=0.0, "Q"=0.0, "Norm  Ampl"=0.0, "z (inf)"=0.0+0.0i, "4corners"={"z (-pi/2)"=0.0+0.0i, "z(inf)"=0.0+0.0i, "z (pi/2)"=0.0+0.0i, "z center"=0.0+0.0i, "z(0)"=0.0+0.0i, "radius"=0.0}}, "timestamp(min)"=1412.7666666656733, "timestamp"=timestamp(3493812587 s since 1904-01-01), "Magn Field(T)"=0.0}, {"temperature"=51.292, "lorentzian"={"Amplitude"=0.0, "omega(0)"=0.0, "Gamma"=0.0, "phase"=0.0, "Q"=0.0, "Norm  Ampl"=0.0, "z (inf)"=0.0+0.0i, "4corners"={"z (-pi/2)"=0.0+0.0i, "z(inf)"=0.0+0.0i, "z (pi/2)"=0.0+0.0i, "z center"=0.0+0.0i, "z(0)"=0.0+0.0i, "radius"=0.0}}, "timestamp(min)"=1414.1000000014901, "timestamp"=timestamp(3493812667 s since 1904-01-01), "Magn Field(T)"=0.0}, {"temperature"=51.226, "lorentzian"={"Amplitude"=0.0, "omega(0)"=0.0, "Gamma"=0.0, "phase"=0.0, "Q"=0.0, "Norm  Ampl"=0.0, "z (inf)"=0.0+0.0i, "4corners"={"z (-pi/2)"=0.0+0.0i, "z(inf)"=0.0+0.0i, "z (pi/2)"=0.0+0.0i, "z center"=0.0+0.0i, "z(0)"=0.0+0.0i, "radius"=0.0}}, "timestamp(min)"=1415.4166666641831, "timestamp"=timestamp(3493812746 s since 1904-01-01), "Magn Field(T)"=0.0}, {"temperature"=51.159, "lorentzian"={"Amplitude"=0.0, "omega(0)"=0.0, "Gamma"=0.0, "phase"=0.0, "Q"=0.0, "Norm  Ampl"=0.0, "z (inf)"=0.0+0.0i, "4corners"={"z (-pi/2)"=0.0+0.0i, "z(inf)"=0.0+0.0i, "z (pi/2)"=0.0+0.0i, "z center"=0.0+0.0i, "z(0)"=0.0+0.0i, "radius"=0.0}}, "timestamp(min)"=1416.75, "timestamp"=timestamp(3493812826 s since 1904-01-01), "Magn Field(T)"=0.0}, {"temperature"=51.091, "lorentzian"={"Amplitude"=0.0, "omega(0)"=0.0, "Gamma"=0.0, "phase"=0.0, "Q"=0.0, "Norm  Ampl"=0.0, "z (inf)"=0.0+0.0i, "4corners"={"z (-pi/2)"=0.0+0.0i, "z(inf)"=0.0+0.0i, "z (pi/2)"=0.0+0.0i, "z center"=0.0+0.0i, "z(0)"=0.0+0.0i, "radius"=0.0}}, "timestamp(min)"=1418.0666666701436, "timestamp"=timestamp(3493812905 s since 1904-01-01), "Magn Field(T)"=0.0}, {"temperature"=51.03, "lorentzian"={"Amplitude"=0.0, "omega(0)"=0.0, "Gamma"=0.0, "phase"=0.0, "Q"=0.0, "Norm  Ampl"=0.0, "z (inf)"=0.0+0.0i, "4corners"={"z (-pi/2)"=0.0+0.0i, "z(inf)"=0.0+0.0i, "z (pi/2)"=0.0+0.0i, "z center"=0.0+0.0i, "z(0)"=0.0+0.0i, "radius"=0.0}}, "timestamp(min)"=1419.3833333328366, "timestamp"=timestamp(3493812984 s since 1904-01-01), "Magn Field(T)"=0.0}, {"temperature"=50.958, "lorentzian"={"Amplitude"=0.0, "omega(0)"=0.0, "Gamma"=0.0, "phase"=0.0, "Q"=0.0, "Norm  Ampl"=0.0, "z (inf)"=0.0+0.0i, "4corners"={"z (-pi/2)"=0.0+0.0i, "z(inf)"=0.0+0.0i, "z (pi/2)"=0.0+0.0i, "z center"=0.0+0.0i, "z(0)"=0.0+0.0i, "radius"=0.0}}, "timestamp(min)"=1420.7166666686535, "timestamp"=timestamp(3493813064 s since 1904-01-01), "Magn Field(T)"=0.0}, {"temperature"=50.9, "lorentzian"={"Amplitude"=0.0, "omega(0)"=0.0, "Gamma"=0.0, "phase"=0.0, "Q"=0.0, "Norm  Ampl"=0.0, "z (inf)"=0.0+0.0i, "4corners"={"z (-pi/2)"=0.0+0.0i, "z(inf)"=0.0+0.0i, "z (pi/2)"=0.0+0.0i, "z center"=0.0+0.0i, "z(0)"=0.0+0.0i, "radius"=0.0}}, "timestamp(min)"=1422.0333333313465, "timestamp"=timestamp(3493813143 s since 1904-01-01), "Magn Field(T)"=0.0}, {"temperature"=50.832, "lorentzian"={"Amplitude"=0.0, "omega(0)"=0.0, "Gamma"=0.0, "phase"=0.0, "Q"=0.0, "Norm  Ampl"=0.0, "z (inf)"=0.0+0.0i, "4corners"={"z (-pi/2)"=0.0+0.0i, "z(inf)"=0.0+0.0i, "z (pi/2)"=0.0+0.0i, "z center"=0.0+0.0i, "z(0)"=0.0+0.0i, "radius"=0.0}}, "timestamp(min)"=1423.3666666671634, "timestamp"=timestamp(3493813223 s since 1904-01-01), "Magn Field(T)"=0.0}, {"temperature"=50.759, "lorentzian"={"Amplitude"=0.0, "omega(0)"=0.0, "Gamma"=0.0, "phase"=0.0, "Q"=0.0, "Norm  Ampl"=0.0, "z (inf)"=0.0+0.0i, "4corners"={"z (-pi/2)"=0.0+0.0i, "z(inf)"=0.0+0.0i, "z (pi/2)"=0.0+0.0i, "z center"=0.0+0.0i, "z(0)"=0.0+0.0i, "radius"=0.0}}, "timestamp(min)"=1424.683333337307, "timestamp"=timestamp(3493813302 s since 1904-01-01), "Magn Field(T)"=0.0}, {"temperature"=50.695, "lorentzian"={"Amplitude"=0.0, "omega(0)"=0.0, "Gamma"=0.0, "phase"=0.0, "Q"=0.0, "Norm  Ampl"=0.0, "z (inf)"=0.0+0.0i, "4corners"={"z (-pi/2)"=0.0+0.0i, "z(inf)"=0.0+0.0i, "z (pi/2)"=0.0+0.0i, "z center"=0.0+0.0i, "z(0)"=0.0+0.0i, "radius"=0.0}}, "timestamp(min)"=1426.0, "timestamp"=timestamp(3493813381 s since 1904-01-01), "Magn Field(T)"=0.0}, {"temperature"=50.631, "lorentzian"={"Amplitude"=0.0, "omega(0)"=0.0, "Gamma"=0.0, "phase"=0.0, "Q"=0.0, "Norm  Ampl"=0.0, "z (inf)"=0.0+0.0i, "4corners"={"z (-pi/2)"=0.0+0.0i, "z(inf)"=0.0+0.0i, "z (pi/2)"=0.0+0.0i, "z center"=0.0+0.0i, "z(0)"=0.0+0.0i, "radius"=0.0}}, "timestamp(min)"=1427.3333333358169, "timestamp"=timestamp(3493813461 s since 1904-01-01), "Magn Field(T)"=0.0}, {"temperature"=50.566, "lorentzian"={"Amplitude"=0.0, "omega(0)"=0.0, "Gamma"=0.0, "phase"=0.0, "Q"=0.0, "Norm  Ampl"=0.0, "z (inf)"=0.0+0.0i, "4corners"={"z (-pi/2)"=0.0+0.0i, "z(inf)"=0.0+0.0i, "z (pi/2)"=0.0+0.0i, "z center"=0.0+0.0i, "z(0)"=0.0+0.0i, "radius"=0.0}}, "timestamp(min)"=1428.6499999985099, "timestamp"=timestamp(3493813540 s since 1904-01-01), "Magn Field(T)"=0.0}, {"temperature"=50.499, "lorentzian"={"Amplitude"=0.0, "omega(0)"=0.0, "Gamma"=0.0, "phase"=0.0, "Q"=0.0, "Norm  Ampl"=0.0, "z (inf)"=0.0+0.0i, "4corners"={"z (-pi/2)"=0.0+0.0i, "z(inf)"=0.0+0.0i, "z (pi/2)"=0.0+0.0i, "z center"=0.0+0.0i, "z(0)"=0.0+0.0i, "radius"=0.0}}, "timestamp(min)"=1429.9666666686535, "timestamp"=timestamp(3493813619 s since 1904-01-01), "Magn Field(T)"=0.0}, {"temperature"=50.428, "lorentzian"={"Amplitude"=0.0, "omega(0)"=0.0, "Gamma"=0.0, "phase"=0.0, "Q"=0.0, "Norm  Ampl"=0.0, "z (inf)"=0.0+0.0i, "4corners"={"z (-pi/2)"=0.0+0.0i, "z(inf)"=0.0+0.0i, "z (pi/2)"=0.0+0.0i, "z center"=0.0+0.0i, "z(0)"=0.0+0.0i, "radius"=0.0}}, "timestamp(min)"=1431.3000000044703, "timestamp"=timestamp(3493813699 s since 1904-01-01), "Magn Field(T)"=0.0}, {"temperature"=50.361, "lorentzian"={"Amplitude"=0.0, "omega(0)"=0.0, "Gamma"=0.0, "phase"=0.0, "Q"=0.0, "Norm  Ampl"=0.0, "z (inf)"=0.0+0.0i, "4corners"={"z (-pi/2)"=0.0+0.0i, "z(inf)"=0.0+0.0i, "z (pi/2)"=0.0+0.0i, "z center"=0.0+0.0i, "z(0)"=0.0+0.0i, "radius"=0.0}}, "timestamp(min)"=1432.6166666671634, "timestamp"=timestamp(3493813778 s since 1904-01-01), "Magn Field(T)"=0.0}, {"temperature"=50.295, "lorentzian"={"Amplitude"=0.0, "omega(0)"=0.0, "Gamma"=0.0, "phase"=0.0, "Q"=0.0, "Norm  Ampl"=0.0, "z (inf)"=0.0+0.0i, "4corners"={"z (-pi/2)"=0.0+0.0i, "z(inf)"=0.0+0.0i, "z (pi/2)"=0.0+0.0i, "z center"=0.0+0.0i, "z(0)"=0.0+0.0i, "radius"=0.0}}, "timestamp(min)"=1433.9500000029802, "timestamp"=timestamp(3493813858 s since 1904-01-01), "Magn Field(T)"=0.0}, {"temperature"=50.232, "lorentzian"={"Amplitude"=0.0, "omega(0)"=0.0, "Gamma"=0.0, "phase"=0.0, "Q"=0.0, "Norm  Ampl"=0.0, "z (inf)"=0.0+0.0i, "4corners"={"z (-pi/2)"=0.0+0.0i, "z(inf)"=0.0+0.0i, "z (pi/2)"=0.0+0.0i, "z center"=0.0+0.0i, "z(0)"=0.0+0.0i, "radius"=0.0}}, "timestamp(min)"=1435.2666666656733, "timestamp"=timestamp(3493813937 s since 1904-01-01), "Magn Field(T)"=0.0}, {"temperature"=50.162, "lorentzian"={"Amplitude"=0.0, "omega(0)"=0.0, "Gamma"=0.0, "phase"=0.0, "Q"=0.0, "Norm  Ampl"=0.0, "z (inf)"=0.0+0.0i, "4corners"={"z (-pi/2)"=0.0+0.0i, "z(inf)"=0.0+0.0i, "z (pi/2)"=0.0+0.0i, "z center"=0.0+0.0i, "z(0)"=0.0+0.0i, "radius"=0.0}}, "timestamp(min)"=1436.5833333358169, "timestamp"=timestamp(3493814016 s since 1904-01-01), "Magn Field(T)"=0.0}, {"temperature"=50.094, "lorentzian"={"Amplitude"=0.0, "omega(0)"=0.0, "Gamma"=0.0, "phase"=0.0, "Q"=0.0, "Norm  Ampl"=0.0, "z (inf)"=0.0+0.0i, "4corners"={"z (-pi/2)"=0.0+0.0i, "z(inf)"=0.0+0.0i, "z (pi/2)"=0.0+0.0i, "z center"=0.0+0.0i, "z(0)"=0.0+0.0i, "radius"=0.0}}, "timestamp(min)"=1437.9166666641831, "timestamp"=timestamp(3493814096 s since 1904-01-01), "Magn Field(T)"=0.0}, {"temperature"=50.029, "lorentzian"={"Amplitude"=0.0, "omega(0)"=0.0, "Gamma"=0.0, "phase"=0.0, "Q"=0.0, "Norm  Ampl"=0.0, "z (inf)"=0.0+0.0i, "4corners"={"z (-pi/2)"=0.0+0.0i, "z(inf)"=0.0+0.0i, "z (pi/2)"=0.0+0.0i, "z center"=0.0+0.0i, "z(0)"=0.0+0.0i, "radius"=0.0}}, "timestamp(min)"=1439.2333333343267, "timestamp"=timestamp(3493814175 s since 1904-01-01), "Magn Field(T)"=0.0}, {"temperature"=49.955, "lorentzian"={"Amplitude"=0.0, "omega(0)"=0.0, "Gamma"=0.0, "phase"=0.0, "Q"=0.0, "Norm  Ampl"=0.0, "z (inf)"=0.0+0.0i, "4corners"={"z (-pi/2)"=0.0+0.0i, "z(inf)"=0.0+0.0i, "z (pi/2)"=0.0+0.0i, "z center"=0.0+0.0i, "z(0)"=0.0+0.0i, "radius"=0.0}}, "timestamp(min)"=1440.5500000044703, "timestamp"=timestamp(3493814254 s since 1904-01-01), "Magn Field(T)"=0.0}, {"temperature"=49.895, "lorentzian"={"Amplitude"=0.0, "omega(0)"=0.0, "Gamma"=0.0, "phase"=0.0, "Q"=0.0, "Norm  Ampl"=0.0, "z (inf)"=0.0+0.0i, "4corners"={"z (-pi/2)"=0.0+0.0i, "z(inf)"=0.0+0.0i, "z (pi/2)"=0.0+0.0i, "z center"=0.0+0.0i, "z(0)"=0.0+0.0i, "radius"=0.0}}, "timestamp(min)"=1441.8833333328366, "timestamp"=timestamp(3493814334 s since 1904-01-01), "Magn Field(T)"=0.0}, {"temperature"=49.828, "lorentzian"={"Amplitude"=0.0, "omega(0)"=0.0, "Gamma"=0.0, "phase"=0.0, "Q"=0.0, "Norm  Ampl"=0.0, "z (inf)"=0.0+0.0i, "4corners"={"z (-pi/2)"=0.0+0.0i, "z(inf)"=0.0+0.0i, "z (pi/2)"=0.0+0.0i, "z center"=0.0+0.0i, "z(0)"=0.0+0.0i, "radius"=0.0}}, "timestamp(min)"=1443.2000000029802, "timestamp"=timestamp(3493814413 s since 1904-01-01), "Magn Field(T)"=0.0}, {"temperature"=49.758, "lorentzian"={"Amplitude"=0.0, "omega(0)"=0.0, "Gamma"=0.0, "phase"=0.0, "Q"=0.0, "Norm  Ampl"=0.0, "z (inf)"=0.0+0.0i, "4corners"={"z (-pi/2)"=0.0+0.0i, "z(inf)"=0.0+0.0i, "z (pi/2)"=0.0+0.0i, "z center"=0.0+0.0i, "z(0)"=0.0+0.0i, "radius"=0.0}}, "timestamp(min)"=1444.5166666656733, "timestamp"=timestamp(3493814492 s since 1904-01-01), "Magn Field(T)"=0.0}, {"temperature"=49.694, "lorentzian"={"Amplitude"=0.0, "omega(0)"=0.0, "Gamma"=0.0, "phase"=0.0, "Q"=0.0, "Norm  Ampl"=0.0, "z (inf)"=0.0+0.0i, "4corners"={"z (-pi/2)"=0.0+0.0i, "z(inf)"=0.0+0.0i, "z (pi/2)"=0.0+0.0i, "z center"=0.0+0.0i, "z(0)"=0.0+0.0i, "radius"=0.0}}, "timestamp(min)"=1445.8500000014901, "timestamp"=timestamp(3493814572 s since 1904-01-01), "Magn Field(T)"=0.0}, {"temperature"=49.627, "lorentzian"={"Amplitude"=0.0, "omega(0)"=0.0, "Gamma"=0.0, "phase"=0.0, "Q"=0.0, "Norm  Ampl"=0.0, "z (inf)"=0.0+0.0i, "4corners"={"z (-pi/2)"=0.0+0.0i, "z(inf)"=0.0+0.0i, "z (pi/2)"=0.0+0.0i, "z center"=0.0+0.0i, "z(0)"=0.0+0.0i, "radius"=0.0}}, "timestamp(min)"=1447.1666666641831, "timestamp"=timestamp(3493814651 s since 1904-01-01), "Magn Field(T)"=0.0}, {"temperature"=49.555, "lorentzian"={"Amplitude"=0.0, "omega(0)"=0.0, "Gamma"=0.0, "phase"=0.0, "Q"=0.0, "Norm  Ampl"=0.0, "z (inf)"=0.0+0.0i, "4corners"={"z (-pi/2)"=0.0+0.0i, "z(inf)"=0.0+0.0i, "z (pi/2)"=0.0+0.0i, "z center"=0.0+0.0i, "z(0)"=0.0+0.0i, "radius"=0.0}}, "timestamp(min)"=1448.5, "timestamp"=timestamp(3493814731 s since 1904-01-01), "Magn Field(T)"=0.0}, {"temperature"=49.488, "lorentzian"={"Amplitude"=0.0, "omega(0)"=0.0, "Gamma"=0.0, "phase"=0.0, "Q"=0.0, "Norm  Ampl"=0.0, "z (inf)"=0.0+0.0i, "4corners"={"z 
